vi "TP1.vi"() -> ()   [LabVIEW 2019]
uses:
  <vilib>/rvi/Emulation/niFpgaGetClockAttributes.vi
  <vilib>/rvi/Emulation/niFpgaSctlEmulationGetInTimedLoop.vi
  <vilib>/rvi/Emulation/niFpgaEmulationReportErrorSimple.vi
  <vilib>/rvi/eio/common/nirviEmuTemplateMethod_errors.vi
  <vilib>/rvi/Emulation/niFpgaCriticalErrorInLSC.vi
  <vilib>/eio/EIONode/EIONode.xnode
panel:
  in  "Reset Button":bool
  out "x+y":u16
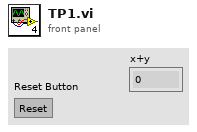
[diagram p1: front panel]
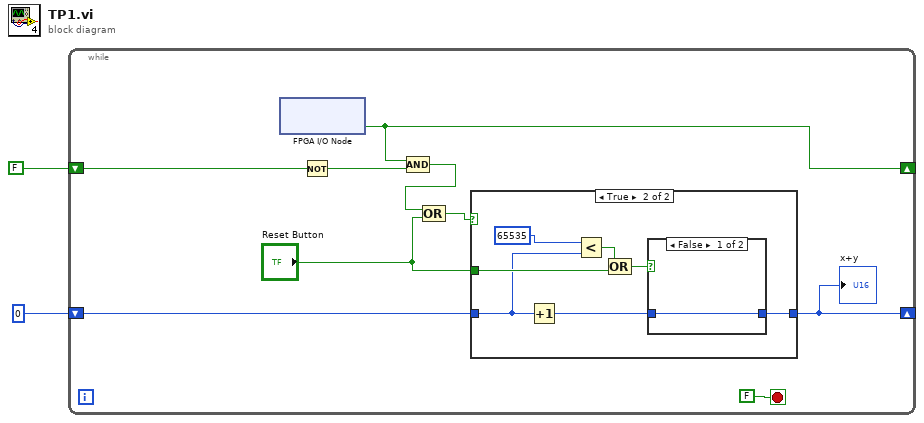
[diagram p0: block diagram]
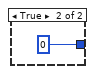
[diagram p3: hidden frame]
diagram:
  n1 = while {
    shift-right: [w6] -> _
    shift-left: u16 0 -> [w10]
    shift-right: [w9] -> _
    shift-left: FALSE -> [w7]
    stop <- FALSE stop-if-true
    n2 = xnode "FPGA I/O Node"() -> ("Button0"=w9:bool)  [unwired: 1 in, 1 out]
    n3 = Not(x=w7) -> (.not. x?=w8:bool)
    n4 = Compound Arithmetic op=AND(w9, w8) -> (w5:bool)
    n5 = Compound Arithmetic op=OR(w5, "Reset Button") -> (w4:bool)
    n6 = case shown="True" w4 {
      tunnel: w10 -> [w12 w14]
      tunnel: [w12 w18] -> w6
      tunnel: "Reset Button" -> [_ w17]
      frame False {
      }
      frame True {
        n7 = Increment(x=w14) -> (x+1=w19:u16)
        n8 = Less?(x=u16 65535, y=w14) -> (x < y?=w15:bool)
        n9 = Compound Arithmetic op=OR(w15, w17) -> (w16:bool)
        n10 = case shown="False" w16 {
          tunnel: w19 -> [w20 _]
          tunnel: [w20 i16 0] -> w18
          frame False {
          }
          frame True {
          }
        }
      }
    }
    "x+y" <- w6
  }
